vi "WavetoXYData(DBL).vi"(8 "error in (no error)":errorcluster caption="エラー入力（エラーなし）", 11 "WaveForm":waveform(dbl)) -> (0 "error out":errorcluster caption="エラー出力", 3 "XY Cluster":cluster{"X":dbl[], "Y":dbl[]})   [LabVIEW 2014]
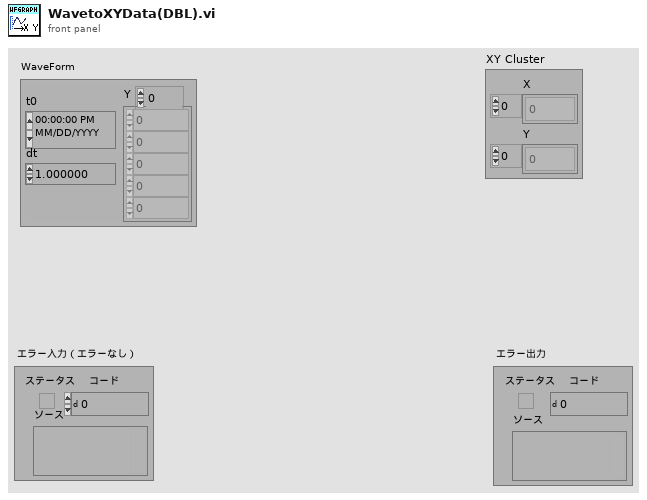
[diagram p1: front panel]
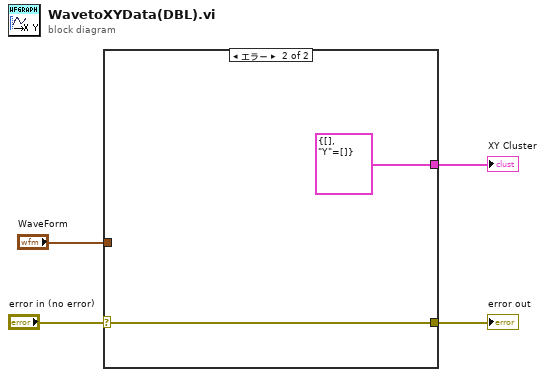
[diagram p0: block diagram]
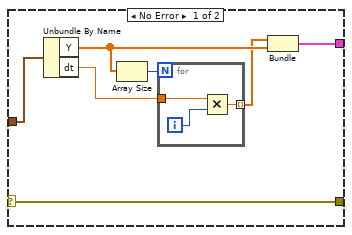
[diagram p2: hidden frame]
diagram:
  n1 = case shown="エラー" "error in (no error)" {
    selector: "error in (no error)" -> [w9 w16]
    tunnel: [w9 w16] -> w3
    tunnel: "WaveForm" -> [w11 _]
    tunnel: [w5 cluster{dbl[], "Y":dbl[]} {[], "Y"=[]}] -> w1
    frame No Error {
      n2 = Unbundle By Name(w11) -> ("Y"=w7:dbl[], "dt"=w10:dbl)
      n3 = Array Size(array=w7) -> (size(s)=w8:i32)
      n4 = for {
        N: w8 -> [_]
        tunnel: w10 -> [w14]
        tunnel: [w12] -> w6 mode=indexing
        i -> [w13]
        n5 = Multiply(x=w14, y=w13) -> (x*y=w12:dbl)
      }
      n6 = Bundle(w6, "Y"=w7) -> (w5:cluster{dbl[], "Y":dbl[]})  [unwired: 1 in]
    }
    frame Error {
    }
  }
  "error out" <- w3
  "XY Cluster" <- w1
